vi "Test_lowerStop.vi"() -> ()   [LabVIEW 2016]
uses:
  Classes/Controllers/I-O/Copy of NI-DAQ Folder/NI-DAQ.lvclass
  D:/INTT/V1/Classes/Controllers/I-O/Copy of I-O Folder/I-O.lvclass
  <vilib>/Utility/file.llb/Read Delimited Spreadsheet (DBL).vi
  Classes/Controllers/Motion/Copy of Motion Folder/Motion.lvclass
  Classes/Controllers/Camera/Copy of Controller Folder/Controller.lvclass
  Classes/Controllers/I-O/Copy of I-O Folder/I-O.lvclass
panel:
  out "x+y":dbl[](array[numeric])
  in  "Parking position":dbl[](array[numeric])=[27.92, 940.1349, 41.7586, -0.0547592]
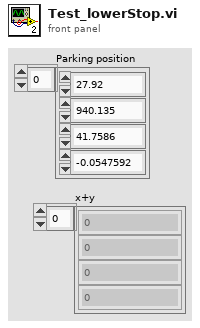
[diagram p1: front panel]
types:
  T1 = typedef "Controller.lvclass/Controllers.ctl" = cluster{"Copy of Motion.lvclass":refnum<class "Motion.lvclass">, "Copy of I-O.lvclass":refnum<class "I-O.lvclass">, "Copy of Dispenser.lvclass":refnum<class "Dispenser.lvclass">}
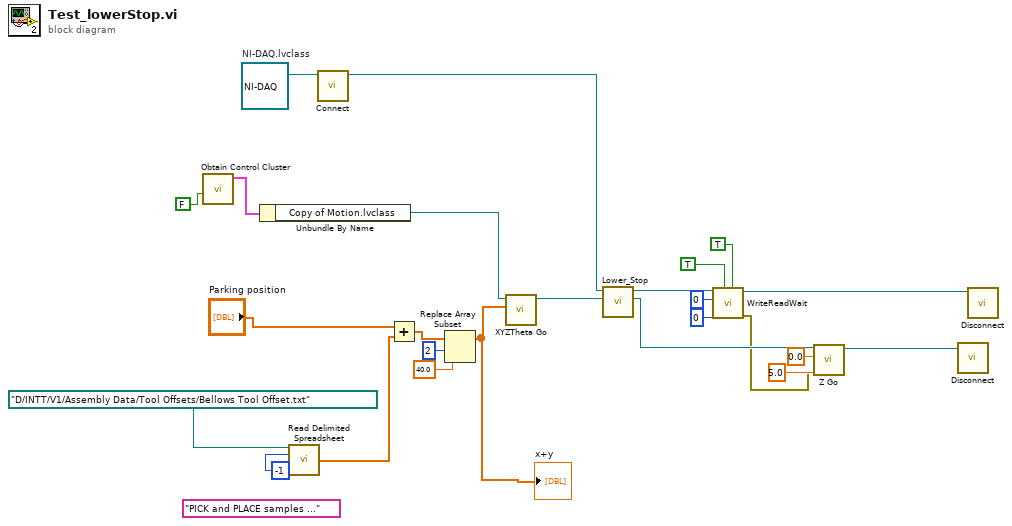
[diagram p0: block diagram]
diagram:
  (unwired) "PICK and PLACE samples ..." ("String")
  w10 = refnum<class "NI-DAQ.lvclass"> refnum  # NI-DAQ.lvclass
  n1 = call "Obtain Control Cluster.vi"("I/O"=FALSE) -> ("Control Out"=w24:T1)  [unwired: 10 in]
  n2 = Unbundle By Name(w24) -> ("Copy of Motion.lvclass"=w23:refnum<class "Motion.lvclass">)
  n3 = call-poly <vilib>:"Read Delimited Spreadsheet.vi"("file path (dialog if empty)"=path "D:/INTT/V1/Assembly Data/Tool Offsets/Bellows Tool Offset.txt", "number of rows (all:-1)"=-1) -> ("first row"=w6:dbl[])  [unwired: 8 in, 5 out]
  n4 = call-dynamic "Connect.vi"("NI-DAQ in"=w10) -> ("NI-DAQ out"=w9:refnum<class "NI-DAQ.lvclass">)  [unwired: 9 in, 1 out]
  n5 = Add(x="Parking position", y=w6) -> (x+y=w4:dbl[])
  n6 = Replace Array Subset(array=w4, new element=40.0 ("new element/subarray"), index=2) -> (w1:dbl[])
  "x+y" <- w1
  n7 = call "XYZTheta Go.vi"("XYZTheta In"=w1, "Motion in"=w23) -> ("Motion out"=w22:refnum<class "Motion.lvclass">)  [unwired: 7 in, 2 out]
  n8 = call "Lower_Stop.vi"("Motion in"=w22, "I-O in"=w9) -> ("Motion out"=w16:refnum<class "Motion.lvclass">, "I-O out"=w19:refnum<class "NI-DAQ.lvclass">)  [unwired: 8 in]
  n9 = call "WriteReadWait.vi"("Read Value"=TRUE, "Write Value"=TRUE, "Read"=0, "Write"=0, "I-O in"=w19) -> ("error out"=w13:errorcluster, "I-O out"=w11:refnum<class "NI-DAQ.lvclass">)  [unwired: 5 in]
  n10 = call-dynamic "Z Go.vi"("error in (no error)"=w13, "Speed"=5.0, "Position"=0.0, "Motion in"=w16) -> ("Motion out"=w12:refnum<class "Motion.lvclass">)  [unwired: 6 in, 1 out]
  n11 = call-dynamic "Disconnect.vi"("Controller in"=w12) -> ()  [unwired: 9 in, 1 out]
  n12 = call-dynamic "Disconnect.vi"("I-O in"=w11) -> ()  [unwired: 9 in, 1 out]
